vi "Lab04.vi"() -> ()   [LabVIEW 2022 SP3]
uses:
  <vilib>/measure/NI_MABase.lvlib
panel:
  out "Waveform Graph 2":dbl[](graph)
  in  "Number of Waves":i32
  out "Waveform Graph":waveform(dbl)[](graph)
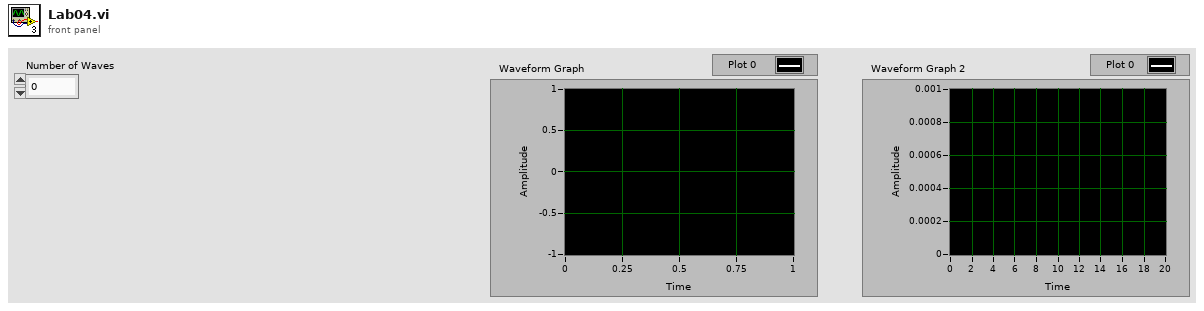
[diagram p1: front panel]
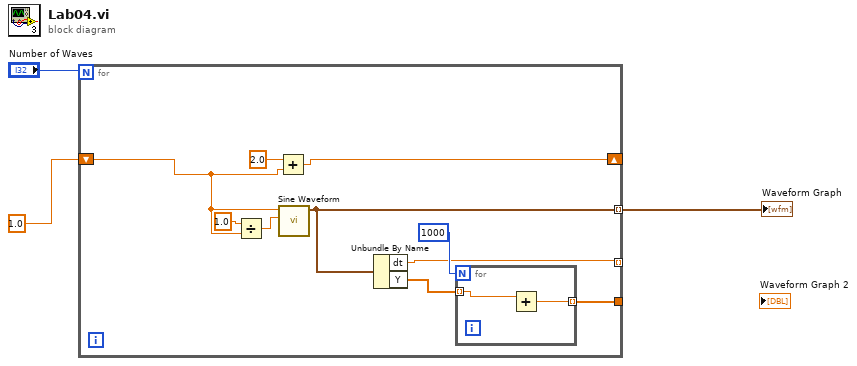
[diagram p0: block diagram]
diagram:
  n1 = for {
    N: "Number of Waves" -> [_]
    shift-right: [w11] -> _
    shift-left: 1.0 -> [w9]
    tunnel: [w10] -> w1 mode=indexing
    tunnel: [w4] -> _ mode=indexing
    tunnel: [w6] -> _
    n2 = Divide(x=1.0, y=w9) -> (x/y=w12:dbl)
    n3 = Add(x=2.0, y=w9) -> (x+y=w11:dbl)
    n4 = call <vilib>:"Sine Waveform.vi"("amplitude"=w12, "frequency"=w9) -> ("signal out"=w10:waveform(dbl))  [unwired: 8 in, 1 out]
    n5 = Unbundle By Name(w10) -> ("dt"=w4:dbl, "Y"=w7:dbl[])
    n6 = for {
      N: 1000 -> [_]
      tunnel: w7 -> [w14] mode=indexing
      tunnel: [w15] -> w6 mode=indexing
      n7 = Add(x=w14) -> (x+y=w15:dbl)  [unwired: 1 in]
    }
  }
  "Waveform Graph" <- w1
